vi "Create Project.vi"(8 "error in (no error)":errorcluster, 9 "Description":string, 10 "Name":string, 11 "Asana in":refnum<class "Asana.lvclass">) -> (0 "error out":errorcluster, 2 "gid":string, 3 "Asana out":refnum<class "Asana.lvclass">)   [LabVIEW 2016, in "Asana.lvclass"]
uses:
  levylab_expt_transport/src/Control Experiment/subVIs/Asana/Asana.lvclass
  levylab_expt_transport/src/Control Experiment/subVIs/Asana/Asana.lvclass/Asana.ctl
  <vilib>/addons/_JKI.lib/REST Client/classes/REST Client/REST Client.lvclass
  <vilib>/addons/_JKI.lib/Serialization/JSON/JKI JSON Serialization.lvlib
panel:
  out "Response body":string
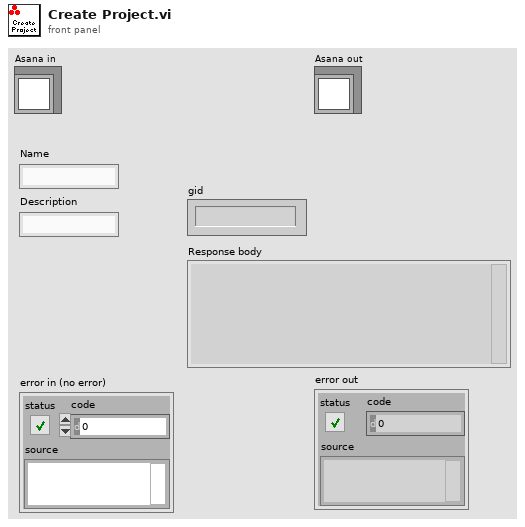
[diagram p1: front panel]
types:
  T1 = typedef "REST Client.lvlib/REST Client.lvclass/HTTP Header.ctl" = cluster{"header":string, "value":string}
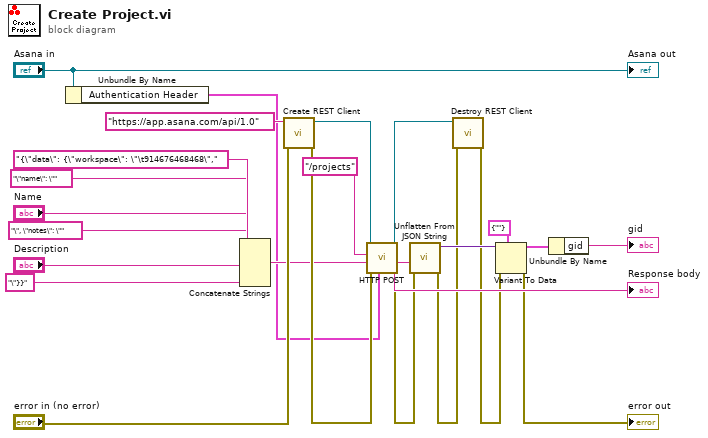
[diagram p0: block diagram]
diagram:
  n1 = Unbundle By Name("Asana in") -> ("Authentication Header"=w2:T1[])
  n2 = Concatenate Strings("{\"data\": {\"workspace\": \"\t914676468468\",", "\"name\": \"" ("string"), "Name", "\", \"notes\": \"" ("string"), "Description", "\"}}" ("string")) -> (w18:string)
  n3 = call <vilib>:"Create REST Client.vi"("error in (no error)"="error in (no error)", "Base URL"="https://app.asana.com/api/1.0") -> ("error out"=w19:errorcluster, "REST Client out"=w23:refnum<class "REST Client.lvclass">)  [unwired: 8 in]
  n4 = call-dynamic "HTTP POST.vi"("request specific headers"=w2, "error in (no error)"=w19, "Request body"=w18, "Path"="/projects", "REST Client in"=w23) -> ("error out"=w15:errorcluster, "Response body"=w16:string, "REST Client out"=w22:refnum<class "REST Client.lvclass">)  [unwired: 1 in, 3 out]
  "Response body" <- w16
  n5 = call <vilib>:"Unflatten From JSON String.vi"("error in (no error)"=w15, "JSON String"=w16) -> ("error out"=w14:errorcluster, "Variant"=w17:variant)  [unwired: 8 in]
  n6 = call-dynamic "Destroy REST Client.vi"("error in (no error)"=w14, "REST Client in"=w22) -> ("error out"=w13:errorcluster)  [unwired: 9 in]
  n7 = Variant To Data(error in=w13, type=cluster{"gid":string} {"gid"=""}, Variant=w17) -> (data=w10:cluster{"gid":string}, error out=→"error out":errorcluster)
  n8 = Unbundle By Name(w10) -> ("gid"=→"gid":string)
  "Asana out" <- "Asana in"
